vi "Reset.vi"(8 "error in (no error)":errorcluster, 11 "Calibrator in":refnum<class "Calibrator.lvclass">) -> (0 "error out":errorcluster, 3 "Calibrator out":refnum<class "Calibrator.lvclass">)   [LabVIEW 2015, in "Calibrator.lvclass"]
uses:
  Calibrator.lvclass
  <instrlib>/Fluke 5XXX Series Multicalibrators/Fluke 5XXX Series Multicalibrators.lvlib
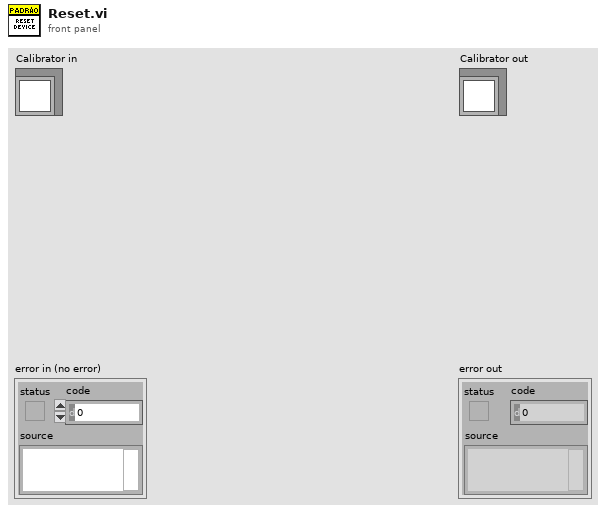
[diagram p1: front panel]
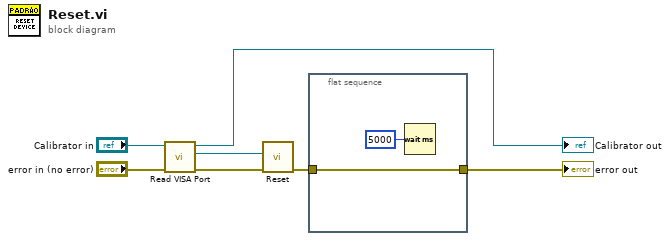
[diagram p0: block diagram]
diagram:
  n1 = call-dynamic "Read VISA Port.vi"("error in (no error)"="error in (no error)", "Device in"="Calibrator in") -> ("error out"=w5:errorcluster, "VISA Port"=w4:refnum<visa-resource-name>, "Device out"=→"Calibrator out":refnum<class "Calibrator.lvclass">)  [unwired: 7 in]
  n2 = call <instrlib>:"Reset.vi"("VISA resource name"=w4, "error in (no error)"=w5) -> ("error out"=w2:errorcluster)  [unwired: 12 in, 1 out]
  n3 = flat-sequence {
    tunnel: w2 -> [w9]
    tunnel: [w9] -> w1
    frame #0 {
      n4 = Wait (ms)(milliseconds to wait=u32 5000) -> ()  [unwired: 1 out]
    }
  }
  "error out" <- w1
